vi "Read error.vi"(8 "error in (no error)":errorcluster, 11 "Main Class in":refnum<class "Main Class.lvclass">) -> (0 "error out":errorcluster, 2 "error":refnum<vi>, 3 "Main Class out":refnum<class "Main Class.lvclass">)   [LabVIEW 2019, in "Main Class.lvclass"]
uses:
  Main Class.lvclass
  Main Class.lvclass/Main Class.ctl
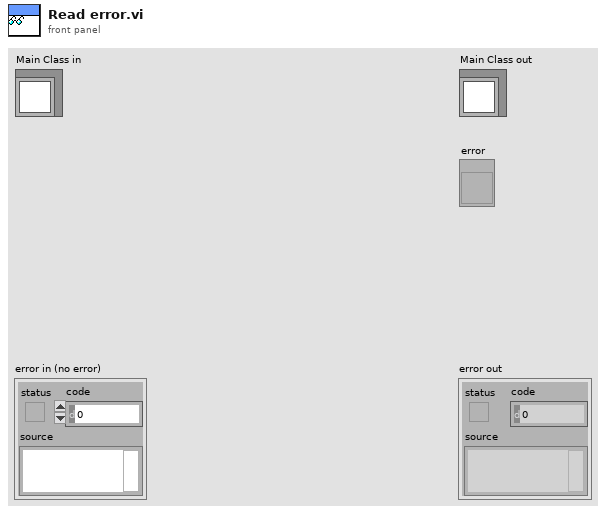
[diagram p1: front panel]
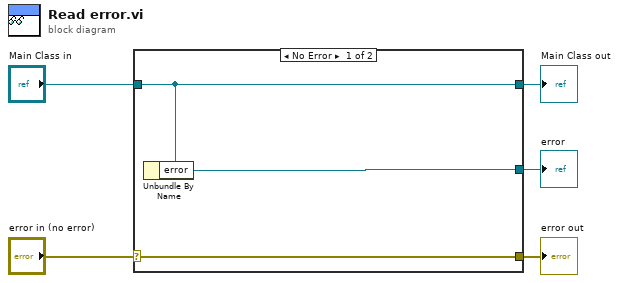
[diagram p0: block diagram]
diagram:
  n1 = case shown="No Error" "error in (no error)" {
    selector: "error in (no error)" -> [w8 w9]
    tunnel: [w8 w9] -> w4
    tunnel: [w7 w10] -> w2
    tunnel: "Main Class in" -> [w7 w10]
    tunnel: [w6 _] -> w1
    frame No Error {
      n2 = Unbundle By Name(w7) -> ("error"=w6:refnum<vi>)
    }
    frame Error {
    }
  }
  "error out" <- w4
  "Main Class out" <- w2
  "error" <- w1
